vi "Stability of Systems.vi"() -> ()   [LabVIEW 2023]
doc: "Displays the amplitude and phase response of the system p(z) = a(z)/b(z) with polynomials a(z) and b(z) determining the stability of the system, where b[0]=1."
uses:
  <vilib>/Analysis/1siggen.llb/Ramp Pattern by Samples.vi
  <vilib>/Analysis/polynomials.llb/Polynomial Roots (DBL).vi
  <vilib>/Analysis/polynomials.llb/1D Rational Polynomial Evaluation (CDB).vi
  <vilib>/Analysis/NI_AALPro.lvlib
  <vilib>/Analysis/NI_AALBase.lvlib
panel:
  in  "Stop":bool
  out "error":i32
  out "system stable?":bool
  out "phase":cluster{"Ramp Pattern":dbl[], dbl[]}(graph)
  out "magnitude":cluster{"Ramp Pattern":dbl[], dbl[]}(graph)
  out "pole zero-plane":cluster{dbl[], dbl[]}[](graph)
  in  "b":dbl[](array[numeric])=[1.0, -1.0, 1.0]
  in  "a":dbl[](array[numeric])=[1.0, 1.1]
  # "Overview: Demonstrates the use of the Polynomial Roots and 1D Rational Polynomial Evaluation VIs to calculate the stability of the system p(z)=b(z)/a(z).\nRequirements: LabVIEW Full Development System\nInstructions:\n1. Run the VI.\n2. Modify the b and a polynomial coefficients and observe the affects on the stability of the system.\n3. Click Stop to stop the VI."
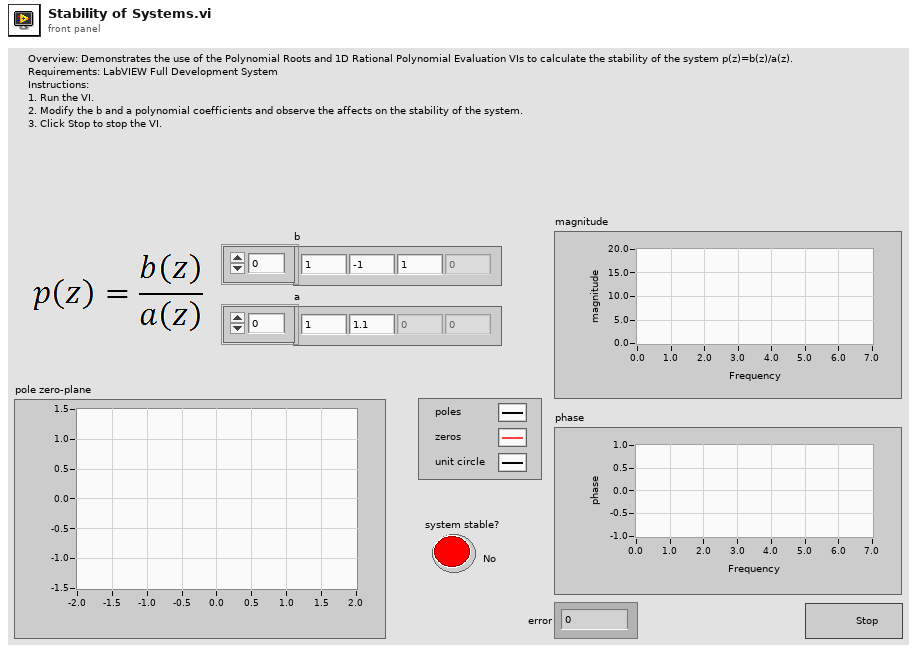
[diagram p1: front panel]
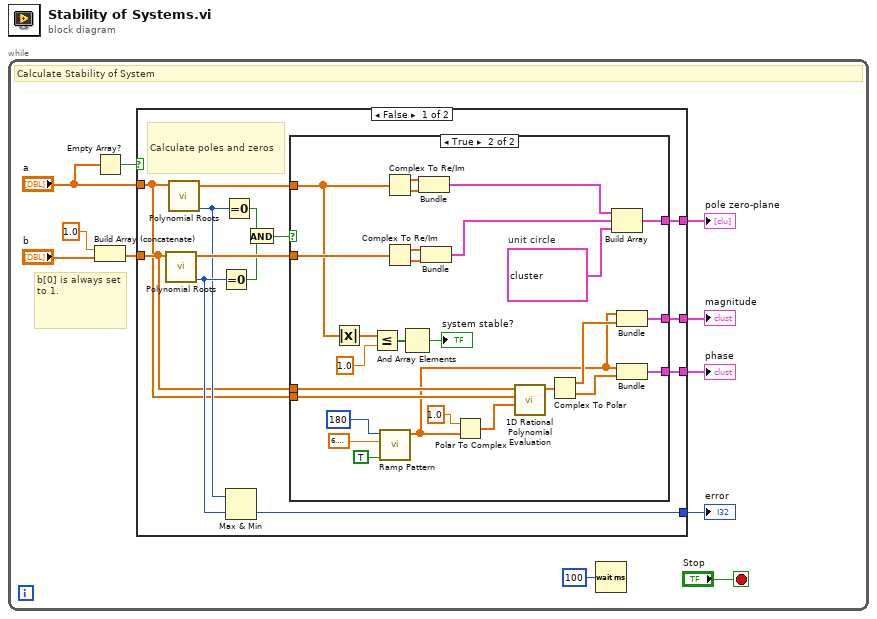
[diagram p0: block diagram]
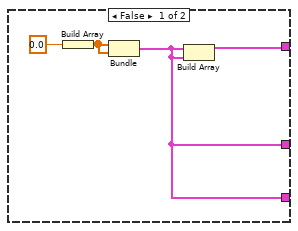
[diagram p2: hidden frame]
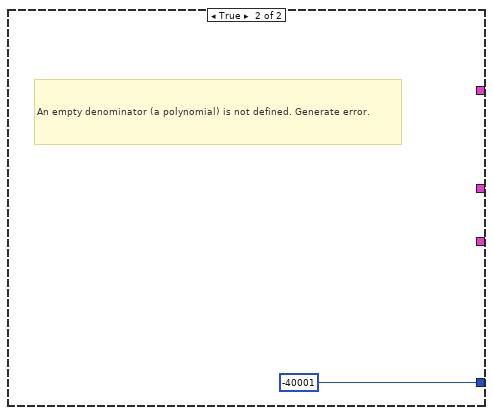
[diagram p3: hidden frame]
diagram:
  n1 = while {
    stop <- "Stop" stop-if-true
    # "b[0] is always set to 1."
    # "Calculate Stability of System"
    n2 = Empty Array?(array="a") -> (empty?=w1:bool)
    n3 = Build Array (concatenate)(1.0, "b") -> (w10:dbl[])
    n4 = case shown="False" w1 {
      tunnel: "a" -> [w12 _]
      tunnel: [w24 _] -> w8
      tunnel: [w23 _] -> w9
      tunnel: w10 -> [w13 _]
      tunnel: [w15 _] -> w7
      tunnel: [w14 -40001] -> w6
      frame False {
        # "Calculate poles and zeros"
        n5 = call-poly <vilib>:"Polynomial Roots.vi"("P(x)"=w13) -> ("error"=w20:i32, "Roots"=w22:cdb[])  [unwired: 9 in]
        n6 = call-poly <vilib>:"Polynomial Roots.vi"("P(x)"=w12) -> ("error"=w19:i32, "Roots"=w21:cdb[])  [unwired: 9 in]
        n7 = Equal To 0?(x=w20) -> (x = 0?=w17:bool)
        n8 = Equal To 0?(x=w19) -> (x = 0?=w16:bool)
        n9 = Max & Min(x=w19, y=w20) -> (min(x,y)=w14:i32)  [unwired: 1 out]
        n10 = And(x=w16, y=w17) -> (x .and. y?=w18:bool)
        n11 = case shown="True" w18 {
          tunnel: w21 -> [_ w33]
          tunnel: w22 -> [_ w55]
          tunnel: w13 -> [_ w37]
          tunnel: w12 -> [_ w36]
          tunnel: [w27 w49] -> w23
          tunnel: [w27 w48] -> w24
          tunnel: [w26 w47] -> w15
          frame False {
            n12 = Build Array(0.0) -> (w28:dbl[])
            n13 = Bundle(w28, w28) -> (w27:cluster{dbl[], dbl[]})  [unwired: 1 in]
            n14 = Build Array(w27, w27) -> (w26:cluster{dbl[], dbl[]}[])
          }
          frame True {
            w34 = cluster{dbl[], dbl[]} {array[1025 elements], array[1025 elements]}  # unit circle
            n15 = Absolute Value(x=w33) -> (abs(x)=w32:dbl[])
            n16 = Less Or Equal?(x=w32, y=1.0) -> (x <= y?=w52:bool[])
            n17 = call-poly <vilib>:"Ramp Pattern.vi"("exclude end?"=TRUE, "end"=6.283185307179586, "samples"=180) -> ("Ramp Pattern"=w30:dbl[])  [unwired: 7 in, 1 out]
            n18 = Complex To Re/Im(x + iy=w33) -> (x=w43:dbl[], y=w54:dbl[])
            n19 = Complex To Re/Im(x + iy=w55) -> (x=w44:dbl[], y=w53:dbl[])
            n20 = And Array Elements(Boolean array=w52) -> (logical AND=→"system stable?":bool)
            n21 = Bundle(w43, w54) -> (w45:cluster{dbl[], dbl[]})  [unwired: 1 in]
            n22 = Bundle(w44, w53) -> (w46:cluster{dbl[], dbl[]})  [unwired: 1 in]
            n23 = Polar To Complex(1:w30, 2:1.0) -> (0:w38:cdb[])
            n24 = call-poly <vilib>:"1D Rational Polynomial Evaluation.vi"("A"=w38, "Q(x)"=w36, "P(x)"=w37) -> ("P(A)/Q(A)"=w35:cdb[])  [unwired: 7 in, 1 out]
            n25 = Complex To Polar(r * e^(i*theta)=w35) -> (r=w51:dbl[], theta=w50:dbl[])
            n26 = Build Array(w45, w46, w34) -> (w47:cluster{dbl[], dbl[]}[])
            n27 = Bundle("Ramp Pattern"=w30, w51) -> (w49:cluster{"Ramp Pattern":dbl[], dbl[]})  [unwired: 1 in]
            n28 = Bundle("Ramp Pattern"=w30, w50) -> (w48:cluster{"Ramp Pattern":dbl[], dbl[]})  [unwired: 1 in]
          }
        }
      }
      frame True {
        # "An empty denominator (a polynomial) is not defined. Generate error."
      }
    }
    "phase" <- w8
    "magnitude" <- w9
    "pole zero-plane" <- w7
    "error" <- w6
    n29 = Wait (ms)(milliseconds to wait=u32 100) -> ()  [unwired: 1 out]
  }
